vi "XY Graph Compute Complex Plot Formula Event.vi"(8 "Error In":errorcluster, 11 "Mouse Click Event Data":T1) -> (0 "Error Out":errorcluster, 1 "Message":string, 2 "Formula":string, 3 "Plot Name":string, 5 "Graph Caption":string)   [LabVIEW 2019, in "XY Graph Add-Ons.lvlib"]
uses:
  XY Graph Add-Ons.lvlib
  XY Graph Mouse Click Event Data.ctl
  XY Graph Refnum.ctl
  <vilib>/Utility/miscctls.llb/LVPoint32TypeDef.ctl
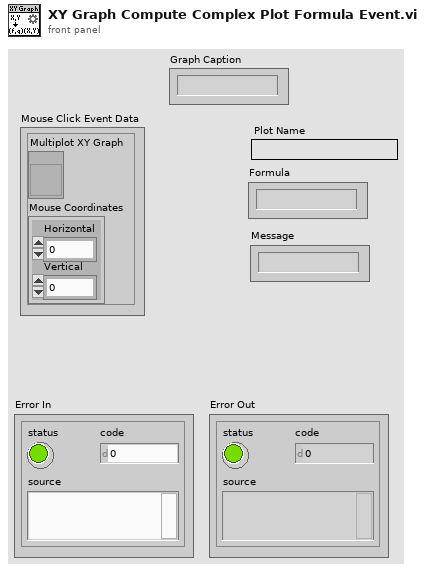
[diagram p1: front panel]
types:
  T1 = typedef "XY Graph Add-Ons.lvlib/XY Graph Mouse Click Event Data.ctl" = cluster{"Multiplot XY Graph":T2, "Mouse Coordinates":T3}
  T2 = typedef "XY Graph Add-Ons.lvlib/XY Graph Refnum.ctl" = refnum<vi>
  T3 = typedef "LVPoint32TypeDef.ctl" = cluster{"Horizontal":i32, "Vertical":i32}
  T4 = cluster{"f(X,Y) Array":dbl[], "g(X,Y) Array":dbl[]}
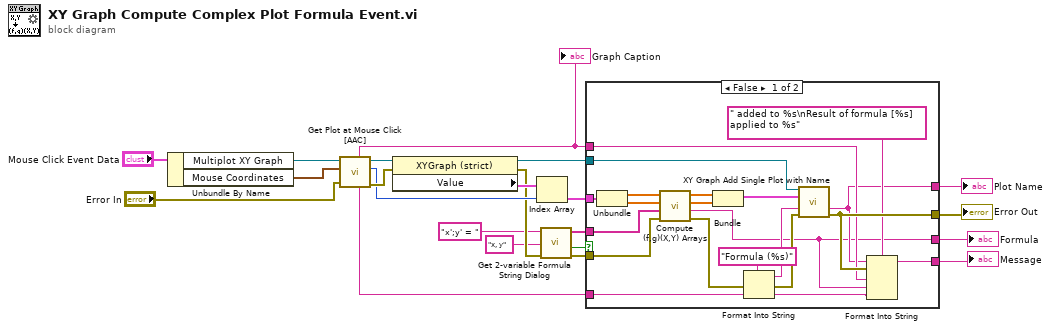
[diagram p0: block diagram]
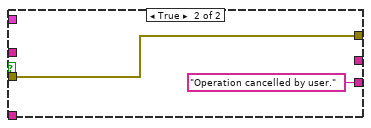
[diagram p2: hidden frame]
diagram:
  n1 = Unbundle By Name("Mouse Click Event Data") -> ("Multiplot XY Graph"=w21:T2, "Mouse Coordinates"=w20:T3)
  n2 = call "Get Plot at Mouse Click [AAC].vi"("error in (no error)"="Error In", "Mouse Click Coordinates"=w20, "XYGraph Ref"=w21) -> ("error out"=w17:errorcluster, "Plot at Coordinates"=w15:i32, "XYGraph Ref"=w18:T2, "Plot Name"=w7:string, "Graph Caption"=w6:string)  [unwired: 2 in, 2 out]
  "Graph Caption" <- w6
  n3 = property class="XYGraph (strict)"(reference=w18, error in=w17) -> (reference out=w10:T2, error out=w14:errorcluster, "Value"=w16:cluster{"X Array":dbl[], "Y Array":dbl[]}[])
  n4 = Index Array(array=w16, index=w15) -> (element=w13:cluster{"X Array":dbl[], "Y Array":dbl[]})
  n5 = call "Get 2-variable Formula String Dialog.vi"("error in (no error)"=w14, "Variables"="x, y", "Formula Names"="x';y' = ") -> ("error out"=w12:errorcluster, "Cancelled?"=w8:bool, "Formula"=w11:string[])  [unwired: 6 in]
  n6 = case shown="False" w8 {
    tunnel: w13 -> [w42 _]
    tunnel: w12 -> [w26 w44]
    tunnel: w11 -> [w24 _]
    tunnel: [w23 _] -> w3
    tunnel: w10 -> [w33 _]
    tunnel: [w38 w44] -> w9
    tunnel: w7 -> [w35 _]
    tunnel: w6 -> [w36 _]
    tunnel: [w34 "Operation cancelled by user."] -> w5
    tunnel: [w32 _] -> w4
    frame False {
      n7 = Unbundle(w42) -> ("X Array"=w31:dbl[], "Y Array"=w30:dbl[])
      n8 = call "Compute (f,g)(X,Y) Arrays.vi"("Error In"=w26, "Formulas"=w24, "Y Array"=w30, "X Array"=w31) -> ("Error Out"=w25:errorcluster, "Formula String"=w23:string, "g(X,Y) Array"=w28:dbl[], "f(X,Y) Array"=w29:dbl[])  [unwired: 4 in]
      n9 = Bundle("f(X,Y) Array"=w29, "g(X,Y) Array"=w28) -> (w27:T4)  [unwired: 1 in]
      n10 = Format Into String(format string="Formula (%s)" ("initial string"), error in=w25, w35) -> (resulting string=w41:string, error out=w40:errorcluster)  [unwired: 1 in]
      n11 = call "XY Graph Add Single Plot with Name.vi"("XYGraph Ref in"=w33, "Plot"=w27, "Plot Name (\"Plot\")"=w41, "error in (no error)"=w40) -> ("Plot Name"=w32:string, "error out"=w38:errorcluster)  [unwired: 8 in, 2 out]
      n12 = Format Into String(format string=" added to %s\nResult of formula [%s] applied to %s", initial string=w32, error in=w38, w36, w23, w35) -> (resulting string=w34:string)  [unwired: 1 out]
    }
    frame True {
    }
  }
  "Error Out" <- w9
  "Formula" <- w3
  "Message" <- w5
  "Plot Name" <- w4
